vi "Write Reply.vi"(8 "error in (no error)":errorcluster, 10 "Reply":string, 11 "GenericCommClass in":refnum<class "ASCIICommClass.lvclass">) -> (0 "error out":errorcluster, 3 "GenericCommClass out":refnum<class "ASCIICommClass.lvclass">)   [LabVIEW 2013, in "ASCIICommClass.lvclass"]
uses:
  ASCIICommClass.lvclass
  ASCIICommClass.lvclass/ASCIICommClass.ctl
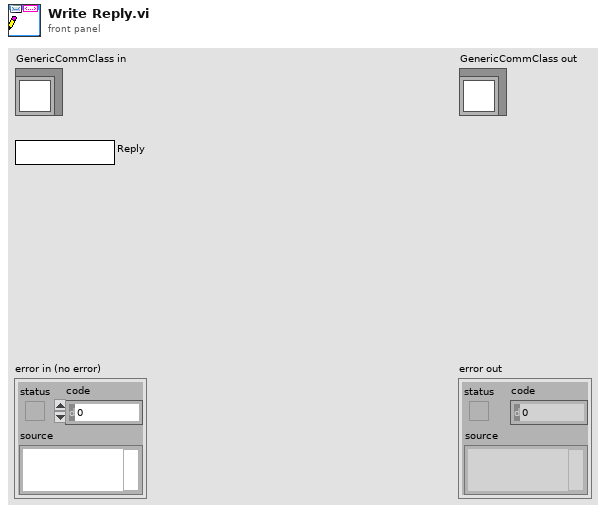
[diagram p1: front panel]
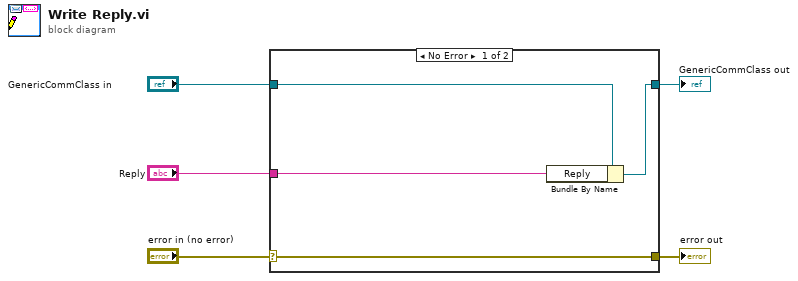
[diagram p0: block diagram]
diagram:
  n1 = case shown="No Error" "error in (no error)" {
    selector: "error in (no error)" -> [w9 w10]
    tunnel: [w9 w10] -> w4
    tunnel: [w7 w11] -> w2
    tunnel: "GenericCommClass in" -> [w8 w11]
    tunnel: "Reply" -> [w6 _]
    frame No Error {
      n2 = Bundle By Name(cluster=w8, "Reply"=w6) -> (w7:refnum<class "ASCIICommClass.lvclass">)
    }
    frame Error {
    }
  }
  "error out" <- w4
  "GenericCommClass out" <- w2
